vi "MartyRequest.vi"(10 "Old Files":T2[](array[typedef])) -> ()   [LabVIEW 2022 SP3]
uses:
  Curtin1_Label.ctl
  <vilib>/Utility/miscctls.llb/LVRangeTypeDef.ctl
panel:
  out "Harmonics":string[][](table)
  out "NewRange":T1
  out "Energy":cluster{"x0":dbl, "df":dbl, dbl[]}[](graph)
  in  "Data Set":u16(ring)
  # "Welcome to Marty's Plots\n\nThese allow one to see the timbre of the note"
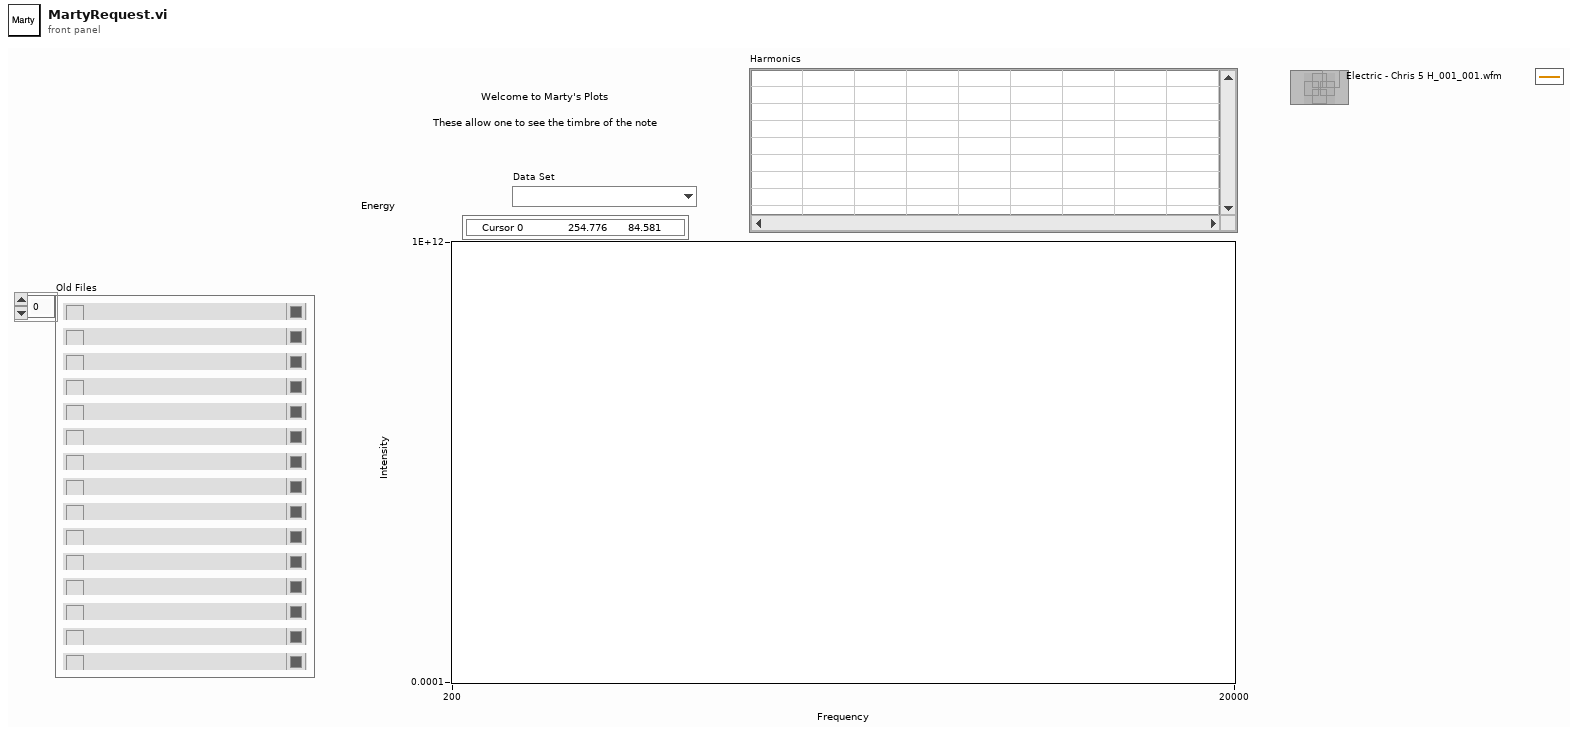
[diagram p1: front panel]
types:
  T1 = typedef "LVRangeTypeDef.ctl" = cluster{"Minimum":dbl, "Maximum":dbl, "Increment":dbl, "Minor Increment":dbl, "Start":dbl}
  T2 = typedef "Curtin1_Label.ctl" = cluster{"Show?":bool, "Name":string, "Color":u32, "Path":path, "Show Notes":bool}
  T3 = cluster{"Start freq":dbl, "Hz resolution":dbl, cdb[]}
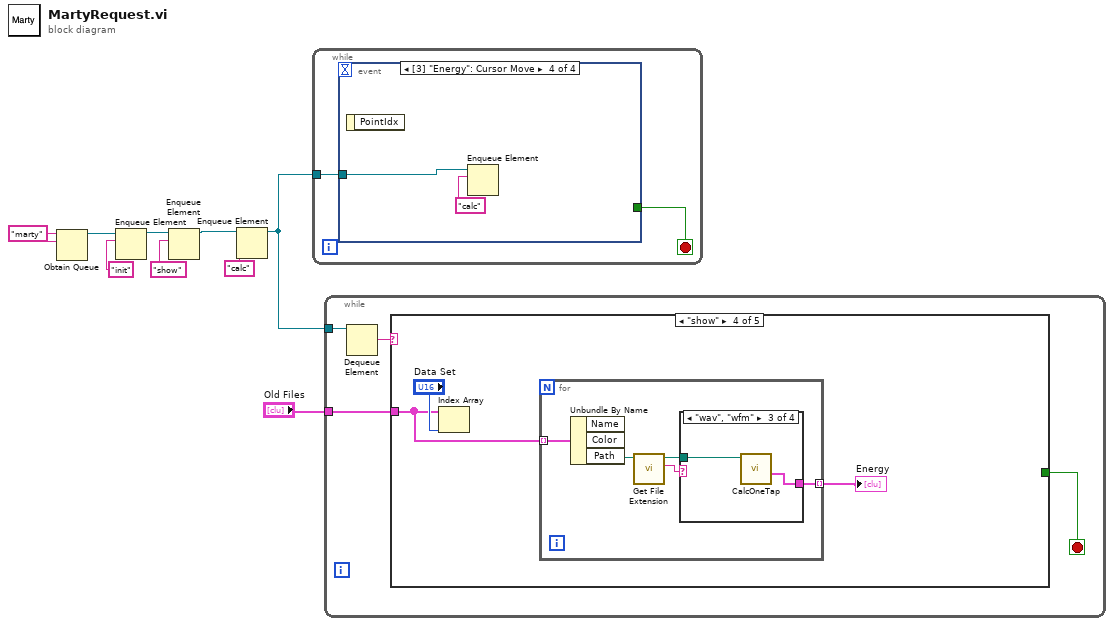
[diagram p0: block diagram]
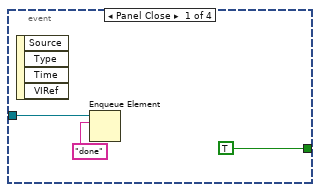
[diagram p2: hidden frame]
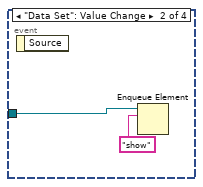
[diagram p3: hidden frame]
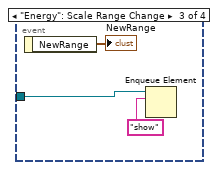
[diagram p4: hidden frame]
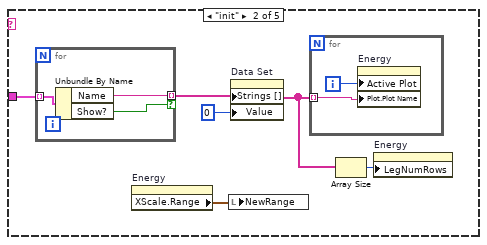
[diagram p6: hidden frame]
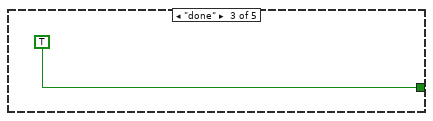
[diagram p7: hidden frame]
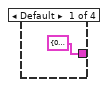
[diagram p8: hidden frame]
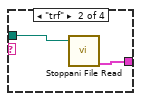
[diagram p9: hidden frame]
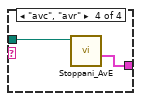
[diagram p10: hidden frame]
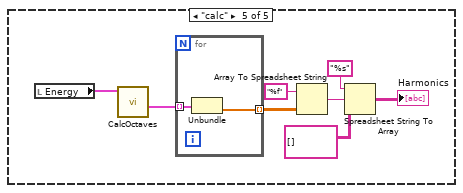
[diagram p11: hidden frame]
diagram:
  w9 = "marty" ("name (unnamed)")
  n1 = Obtain Queue(name (unnamed)=w9, element data type=w9) -> (queue out=w5:refnum<queue>)  [unwired: 3 in, 2 out]
  n2 = Enqueue Element(queue=w5, element="init") -> (queue out=w4:refnum<queue>)  [unwired: 2 in, 2 out]
  n3 = Enqueue Element(queue=w4, element="show") -> (queue out=w2:refnum<queue>)  [unwired: 2 in, 2 out]
  n4 = Enqueue Element(queue=w2, element="calc") -> (queue out=w1:refnum<queue>)  [unwired: 2 in, 2 out]
  n5 = while {
    tunnel: w1 -> [w10]
    stop <- w11 stop-if-true
    n6 = event shown="[3] \"Energy\": Cursor Move" {
      selector: _ -> [_ _ _ _]
      dyn-events: _ -> [_ _ _ _]
      timeout: _ -> [_ _ _ _]
      tunnel: [TRUE _ _ _] -> w11
      tunnel: w10 -> [w12 w15 w18 w20]
      event Panel Close {
        n7 = event-data() -> ()  [unwired: 1 in, 4 out]
        n8 = Enqueue Element(queue=w12, element="done") -> ()  [unwired: 2 in, 3 out]
      }
      event "Data Set": Value Change {
        n9 = event-data() -> ()  [unwired: 1 in, 1 out]
        n10 = Enqueue Element(queue=w15, element="show") -> ()  [unwired: 2 in, 3 out]
      }
      event "Energy": Scale Range Change {
        n11 = event-data() -> ("NewRange"=→"NewRange":T1)  [unwired: 1 in]
        n12 = Enqueue Element(queue=w18, element="show") -> ()  [unwired: 2 in, 3 out]
      }
      event "Energy": Cursor Move {
        n13 = event-data() -> ()  [unwired: 1 in, 1 out]
        n14 = Enqueue Element(queue=w20, element="calc") -> ()  [unwired: 2 in, 3 out]
      }
    }
  }
  n15 = while {
    tunnel: w1 -> [w25]
    tunnel: "Old Files" -> [w22]
    stop <- w23 stop-if-true
    n16 = Dequeue Element(queue=w25) -> (element=w24:string)  [unwired: 2 in, 3 out]
    n17 = case shown="\"show\"" w24 {
      tunnel: [_ _ TRUE _ _] -> w23
      tunnel: w22 -> [_ w30 _ w38 _]
      frame Default {
      }
      frame "init" {
        n18 = for {
          tunnel: w30 -> [w35] mode=indexing
          tunnel: [w34] -> w27 mode=indexing if=w33
          n19 = Unbundle By Name(w35) -> ("Name"=w34:string, "Show?"=w33:bool)
        }
        n20 = property on="Energy" class="WFGraph (strict)"() -> ("XScale.Range"=w28:T1)  [unwired: 2 in, 2 out]
        n21 = local write "NewRange"(w28) -> ()
        n22 = property on="Data Set" class="Ring (strict)"("Strings []"=w27, "Value"=0) -> ()  [unwired: 2 in, 2 out]
        n23 = for {
          tunnel: w27 -> [w31] mode=indexing
          i -> [w32]
          n24 = property on="Energy" class="WFGraph (strict)"("Active Plot"=w32, "Plot.Plot Name"=w31) -> ()  [unwired: 2 in, 2 out]
        }
        n25 = Array Size(array=w27) -> (size(s)=w26:i32)
        n26 = property on="Energy" class="WFGraph (strict)"("LegNumRows"=w26) -> ()  [unwired: 2 in, 2 out]
      }
      frame "done" {
      }
      frame "show" {
        n27 = Index Array(array=w38, index="Data Set") -> ()  [unwired: 1 out]
        n28 = for {
          tunnel: w38 -> [w41] mode=indexing
          tunnel: [w40] -> w37 mode=indexing
          n29 = Unbundle By Name(w41) -> ("Path"=w44:path)  [unwired: 2 out]
          n30 = call <vilib>:"Get File Extension.vi"("file"=w44) -> ("lowercase file extension"=w42:string, "dup file"=w43:path)  [unwired: 6 in, 3 out]
          n31 = case shown="\"wav\", \"wfm\"" w42 {
            tunnel: [T3 {"Start freq"=0.0, "Hz resolution"=0.0, []} ("Waveform Graph") w46 w48 w51] -> w40
            tunnel: w43 -> [_ w47 w49 w50]
            frame Default {
            }
            frame "trf" {
              n32 = call "Stoppani File Read.vi"("String in"=w47) -> ("Complex FRF"=w46:cluster{"t0":dbl, "dt":dbl, "Y":cdb[]})  [unwired: 2 in, 3 out]
            }
            frame "wav", "wfm" {
              n33 = call "CalcOneTap.vi"("wavform file"=w49) -> ("Complex FRF"=w48:cluster{dbl, "df":dbl, cdb[]})  [unwired: 7 in, 3 out]
            }
            frame "avc", "avr" {
              n34 = call "Stoppani_AvE.vi"("file (use dialog)"=w50) -> ("Complex FRF"=w51:cluster{"t0":dbl, "df":dbl, "Y":cdb[]})  [unwired: 7 in, 3 out]
            }
          }
        }
        "Energy" <- w37
      }
      frame "calc" {
        n35 = local read "Energy"() -> (w59:cluster{"x0":dbl, "df":dbl, dbl[]}[])
        n36 = call "CalcOctaves.vi"("Energy"=w59) -> ("XY Graph"=w58:cluster{dbl[], dbl[]}[])  [unwired: 8 in, 2 out]
        n37 = for {
          tunnel: w58 -> [w61] mode=indexing
          tunnel: [w60] -> w57 mode=indexing
          n38 = Unbundle(w61) -> (w60:dbl[])  [unwired: 1 out]
        }
        n39 = Array To Spreadsheet String(array=w57, 3:"%f" ("format string")) -> (spreadsheet string=w55:string)  [unwired: 1 in]
        n40 = Spreadsheet String To Array(format string="%s", spreadsheet string=w55, array type (2D Dbl)=string[][] [] ("Harmonics")) -> (array=→"Harmonics":string[][])  [unwired: 1 in]
      }
    }
  }
